vi "CommonVIs_ListHirearchaRecursive.vi"(1 "FilePath":path, 2 "FileSearchPattern":string, 3 "IgnoreClassMemberVIs(False)":bool, 5 "error in (no error)":errorcluster) -> (16 "Files":path[](array[path]), 17 "VIRefs":refnum<vi>[](array[refnum]), 19 "error out":errorcluster)   [LabVIEW 2020]
doc: "Recursively deletes contents of a directory, including the directory itself as default.\nif <B>deleteTopDirAlso</B> is set to false, the selected directory will not be removed."
panel:
  in  "reference":refnum<vi>
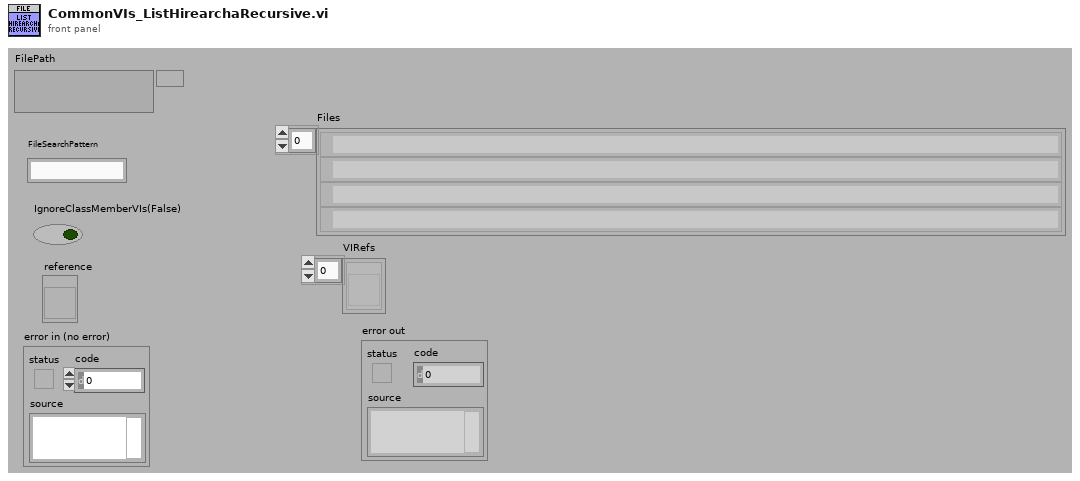
[diagram p1: front panel]
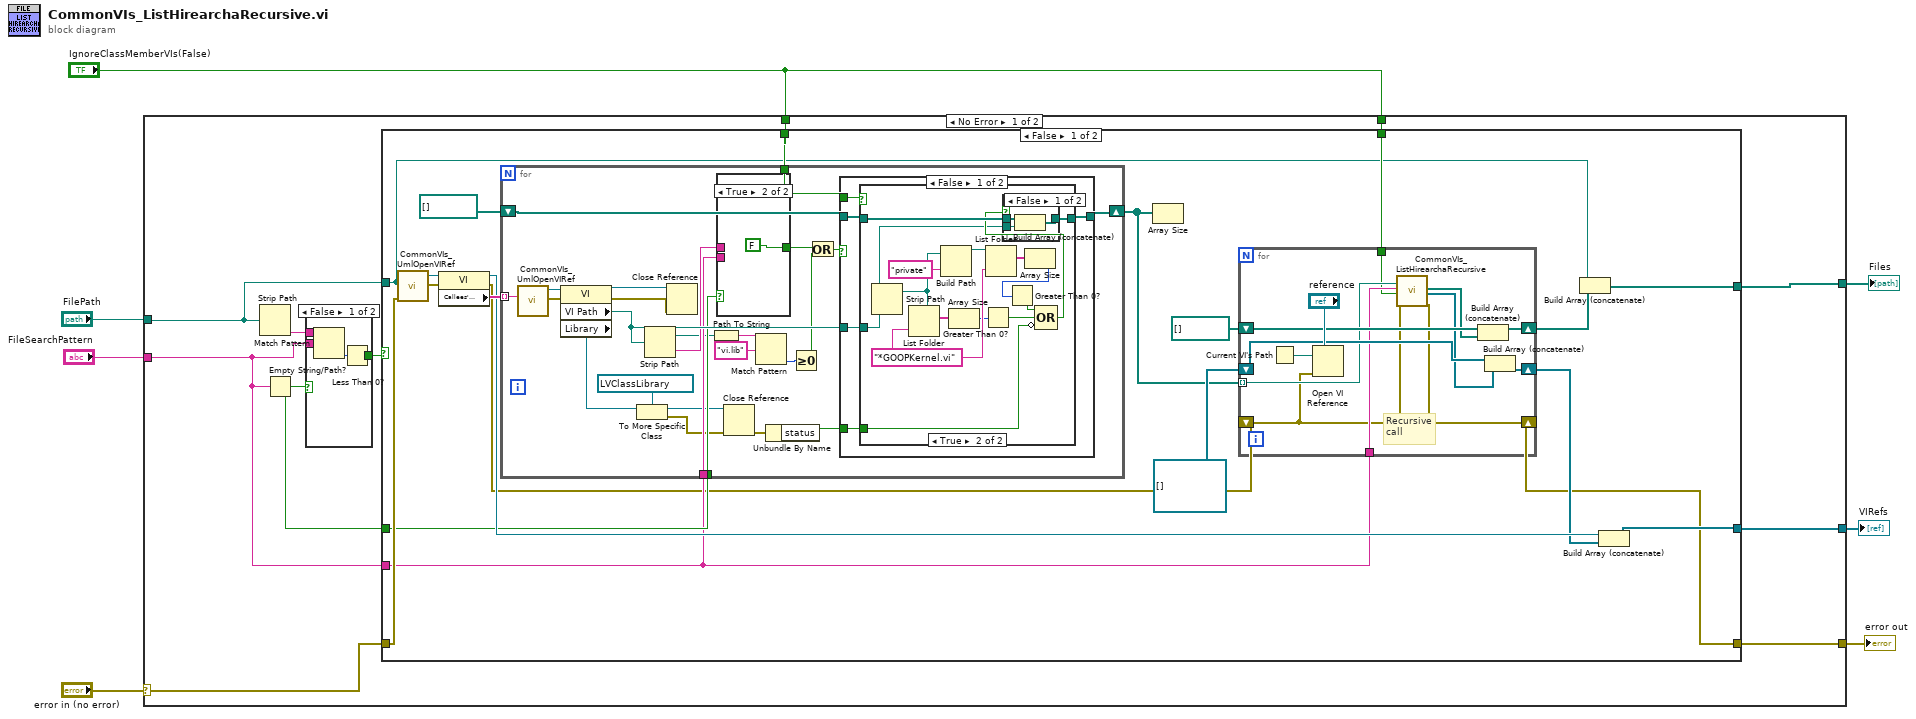
[diagram p0: block diagram]
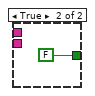
[diagram p2: hidden frame]
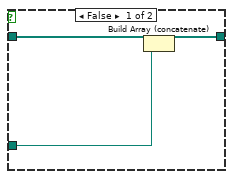
[diagram p3: hidden frame]
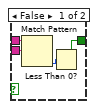
[diagram p6: hidden frame]
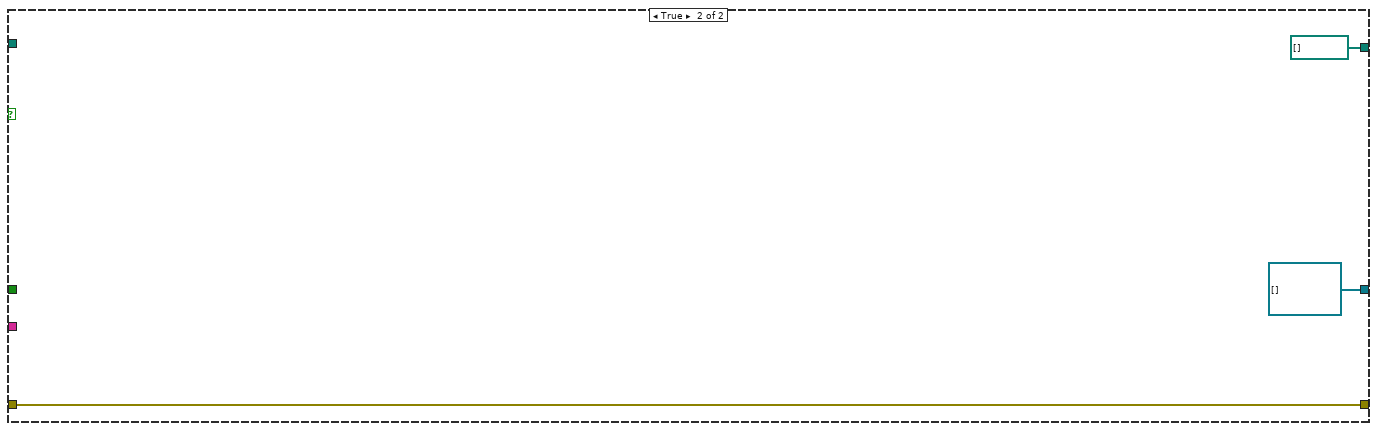
[diagram p7: hidden frame]
diagram:
  n1 = case shown="No Error" "error in (no error)" {
    selector: "error in (no error)" -> [w13 w118]
    tunnel: "FilePath" -> [w12 _]
    tunnel: [w18 w118] -> w6
    tunnel: "FileSearchPattern" -> [w9 _]
    tunnel: [w17 _] -> w3
    tunnel: [w16 _] -> w1
    tunnel: "IgnoreClassMemberVIs(False)" -> [w15 _]
    tunnel: "IgnoreClassMemberVIs(False)" -> [w14 _]
    frame No Error {
      n2 = Strip Path(path=w12) -> (name=w11:string)  [unwired: 1 out]
      n3 = Empty String/Path?(string/path=w9) -> (empty?=w8:bool)
      n4 = case shown="False" w8 {
        tunnel: w11 -> [w22 _]
        tunnel: [w20 FALSE] -> w10
        tunnel: w9 -> [w19 _]
        frame False {
          n5 = Match Pattern(string=w22, regular expression=w19) -> (offset past match=w21:i32)  [unwired: 4 out]
          n6 = Less Than 0?(x=w21) -> (x < 0?=w20:bool)
        }
        frame True {
        }
      }
      n7 = case shown="False" w10 {
        tunnel: [w29 w115] -> w18
        tunnel: [w42 path[] []] -> w17
        tunnel: [w30 refnum<vi>[] [] ("VIRefs")] -> w16
        tunnel: w15 -> [w40 _]
        tunnel: w14 -> [w39 _]
        tunnel: w13 -> [w37 w115]
        tunnel: w12 -> [w28 _]
        tunnel: w9 -> [w26 _]
        tunnel: w8 -> [w27 _]
        frame False {
          n8 = call <resource>:"CommonVIs_UmlOpenVIRef.vi"("error in"=w37, "ViPath/ViName"=w28) -> ("error out"=w36:errorcluster, "vi reference"=w35:refnum<vi>)  [unwired: 2 in, 6 out]
          n9 = property class="VI"(reference=w35, error in=w36) -> (reference out=w33:refnum<vi>, error out=w24:errorcluster, "Callees' Names"=w34:string[])
          n10 = for {
            tunnel: w39 -> [w81]
            shift-right: [w79] -> w25
            shift-left: path[] [] -> [w80]
            tunnel: w34 -> [w78] mode=indexing
            tunnel: w27 -> [w72]
            tunnel: w26 -> [w70]
            n11 = call <resource>:"CommonVIs_UmlOpenVIRef.vi"("ViPath/ViName"=w78) -> ("error out"=w76:errorcluster, "vi reference"=w77:refnum<vi>)  [unwired: 3 in, 6 out]
            n12 = property class="VI"(reference=w77, error in=w76) -> (reference out=w75:refnum<vi>, error out=w74:errorcluster, "VI Path"=w73:path, "Library"=w62:refnum<vi>)
            n13 = To More Specific Class(target class=refnum<vi> refnum ("Library"), reference=w62) -> (specific class reference=w60:refnum<vi>, error out=w59:errorcluster)  [unwired: 1 in]
            n14 = Strip Path(path=w73) -> (stripped path=w67:path, name=w71:string)
            n15 = Close Reference(reference=w75, error in (no error)=w74) -> ()  [unwired: 1 out]
            n16 = Path To String(path=w67) -> (string=w66:string)
            n17 = case shown="True" w72 {
              tunnel: w71 -> [w113 _]
              tunnel: [w111 FALSE] -> w68
              tunnel: w70 -> [w110 _]
              frame False {
                n18 = Match Pattern(string=w113, regular expression=w110) -> (offset past match=w112:i32)  [unwired: 4 out]
                n19 = Less Than 0?(x=w112) -> (x < 0?=w111:bool)
              }
              frame True {
              }
            }
            n20 = Close Reference(reference=w60, error in (no error)=w59) -> (error out=w58:errorcluster)
            n21 = Match Pattern(string=w66, regular expression="vi.lib") -> (offset past match=w64:i32)  [unwired: 4 out]
            n22 = Unbundle By Name(w58) -> ("status"=w57:bool)
            n23 = Greater Or Equal To 0?(x=w64) -> (x >= 0?=w63:bool)
            n24 = Or(x=w68, y=w63) -> (x .or. y?=w69:bool)
            n25 = case shown="False" w69 {
              tunnel: w81 -> [w86 _]
              tunnel: w80 -> [w85 w109]
              tunnel: [w84 w109] -> w79
              tunnel: w73 -> [w83 _]
              tunnel: w57 -> [w82 _]
              frame False {
                n26 = case shown="True" w86 {
                  tunnel: w85 -> [w89 w95]
                  tunnel: [w88 w94] -> w84
                  tunnel: w83 -> [w87 w91]
                  tunnel: w82 -> [_ w90]
                  frame False {
                    n27 = Build Array (concatenate)(w89, w87) -> (w88:path[])
                  }
                  frame True {
                    w102 = "*GOOPKernel.vi" ("pattern")
                    n28 = Strip Path(path=w91) -> (stripped path=w92:path)  [unwired: 1 out]
                    n29 = List Folder(path=w92, pattern=w102) -> (filenames=w101:string[])  [unwired: 1 in, 4 out]
                    n30 = Build Path(base path=w92, name or relative path="private") -> (appended path=w103:path)
                    n31 = Array Size(array=w101) -> (size(s)=w99:i32)
                    n32 = Greater Than 0?(x=w99) -> (x > 0?=w97:bool)
                    n33 = List Folder(path=w103, pattern=w102) -> (filenames=w100:string[])  [unwired: 1 in, 4 out]
                    n34 = Array Size(array=w100) -> (size(s)=w98:i32)
                    n35 = Greater Than 0?(x=w98) -> (x > 0?=w96:bool)
                    n36 = Compound Arithmetic op=OR(w96, w97, invert w90) -> (w93:bool)
                    n37 = case shown="False" w93 {
                      tunnel: w95 -> [w107 w108]
                      tunnel: [w106 w108] -> w94
                      tunnel: w91 -> [w105 _]
                      frame False {
                        n38 = Build Array (concatenate)(w107, w105) -> (w106:path[])
                      }
                      frame True {
                      }
                    }
                  }
                }
              }
              frame True {
              }
            }
          }
          n39 = Array Size(array=w25) -> ()  [unwired: 1 out]
          n40 = for {
            shift-right: [w44] -> w29
            shift-left: w24 -> [w45]
            shift-right: [w54] -> w43
            shift-left: path[] [] -> [w53]
            shift-right: [w51] -> w31
            shift-left: refnum<vi>[] [] ("VIRefs") -> [w52]
            tunnel: w26 -> [w49]
            tunnel: w40 -> [w48]
            tunnel: w25 -> [w50] mode=indexing
            # "Recursive\ncall"
            n41 = Current VI's Path() -> (path=w56:path)
            n42 = Open VI Reference(type specifier VI Refnum (for type only)="reference", vi path=w56, error in (no error)=w45) -> ()  [unwired: 5 out]
            n43 = call <resource>:"CommonVIs_ListHirearchaRecursive.vi"("FilePath"=w50, "FileSearchPattern"=w49, "IgnoreClassMemberVIs(False)"=w48, "error in (no error)"=w45) -> ("Files"=w47:path[], "VIRefs"=w46:refnum<vi>[], "error out"=w44:errorcluster)  [unwired: 13 in]
            n44 = Build Array (concatenate)(w53, w47) -> (w54:path[])
            n45 = Build Array (concatenate)(w52, w46) -> (w51:refnum<vi>[])
          }
          n46 = Build Array (concatenate)(w28, w43) -> (w42:path[])
          n47 = Build Array (concatenate)(w33, w31) -> (w30:refnum<vi>[])
        }
        frame True {
        }
      }
    }
    frame Error {
    }
  }
  "error out" <- w6
  "VIRefs" <- w1
  "Files" <- w3
